vi "Remote Panel Multiple Client.vi"() -> ()   [LabVIEW 2024]
doc: "This VI illustrates how to programmatically connect to a remote front panel. A connection is established to the specified VI and control can also be requested. Once control is requested, the VI can only be run once since the server will close the connection automatically after one run."
panel:
  out "status":bool
  in  "Close Connection":bool
  in  "Open Connection":bool
  in  "Listbox":i32(listbox)
  in  "Stop":bool
  in  "Release Control":bool
  in  "Request Control":bool
  in  "RP Server Port":i32=8000
  in  "RP Server Address":string="localhost"
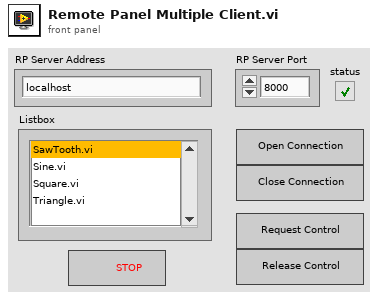
[diagram p1: front panel]
types:
  T1 = enum32{"invalid app kind", "Development System", "Run Time System", "Student Edition", "Embedded LabVIEW", "Evaluation", "Custom"}
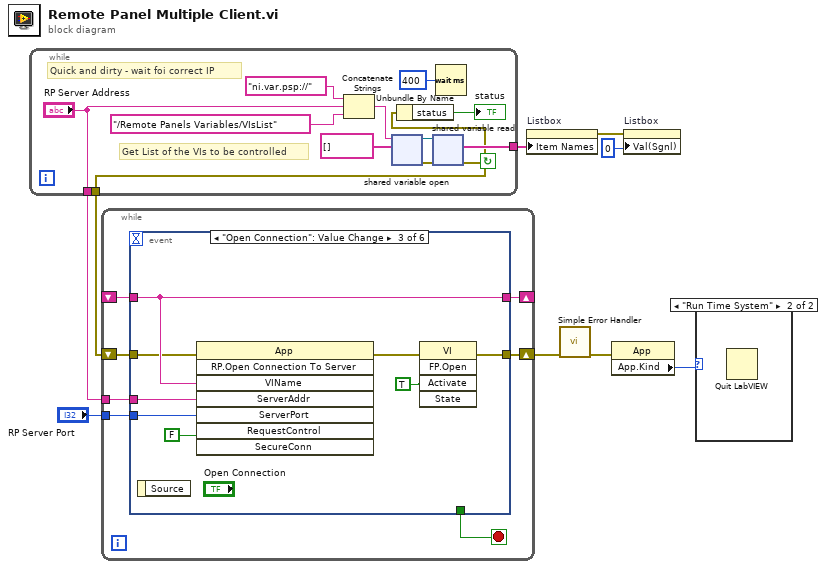
[diagram p0: block diagram]
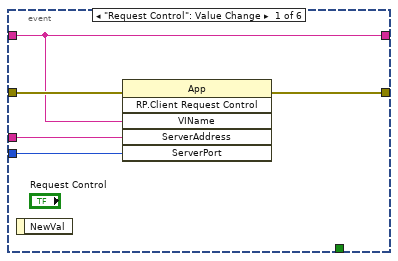
[diagram p3: hidden frame]
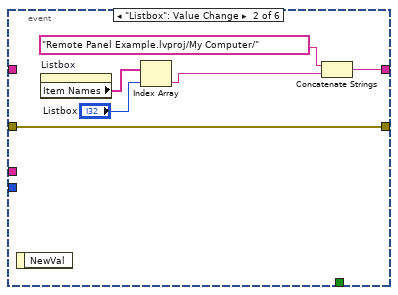
[diagram p4: hidden frame]
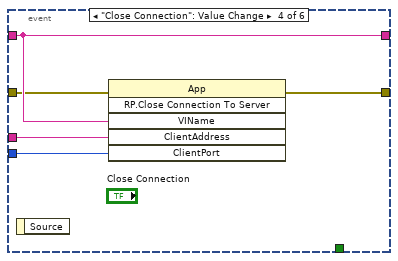
[diagram p5: hidden frame]
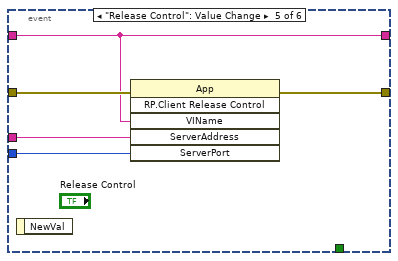
[diagram p6: hidden frame]
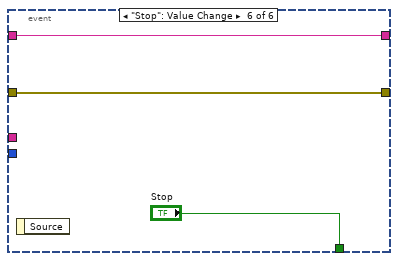
[diagram p7: hidden frame]
diagram:
  n1 = while {
    tunnel: [w17] -> w7
    tunnel: [w11] -> w6
    tunnel: ["RP Server Address"] -> w1
    stop <- w11 continue-if-true
    # "Quick and dirty - wait foi correct IP"
    # "Get List of the VIs to be controlled"
    n2 = Concatenate Strings("ni.var.psp://" ("string"), "RP Server Address", "/Remote Panels Variables/VIsList" ("/Remote Panels Variables/VIsList")) -> (w13:string)
    n3 = shared-variable-open(w13, string[] []) -> (w19:refnum<k21>, w18:errorcluster)  [unwired: 2 in]
    n4 = shared-variable-read(w19, w18) -> (w11:errorcluster, w17:string[])  [unwired: 2 out]
    n5 = Unbundle By Name(w11) -> ("status"=→"status":bool)
    n6 = Wait (ms)(milliseconds to wait=u32 400) -> ()  [unwired: 1 out]
  }
  n7 = while {
    tunnel: "RP Server Port" -> [w26]
    tunnel: w1 -> [w25]
    shift-right: [w27] -> w9
    shift-left: w6 -> [w24]
    shift-right: [w22] -> _
    shift-left: _ -> [w21]
    stop <- w23 stop-if-true
    n8 = event shown="[2] \"Open Connection\": Value Change" {
      selector: _ -> [_ _ _ _ _ _]
      dyn-events: _ -> [_ _ _ _ _ _]
      timeout: _ -> [_ _ _ _ _ _]
      tunnel: w24 -> [w32 w33 w40 w48 w56 w58]
      tunnel: [w31 w33 w39 w47 w55 w58] -> w27
      tunnel: w26 -> [w30 _ w42 w50 w54 _]
      tunnel: w25 -> [w29 _ w43 w51 w53 _]
      tunnel: [_ _ _ _ _ "Stop"] -> w23
      tunnel: [w28 w34 w41 w49 w52 w57] -> w22
      tunnel: w21 -> [w28 _ w41 w49 w52 w57]
      event "Request Control": Value Change {
        n9 = event-data() -> ()  [unwired: 1 in, 1 out]
        n10 = invoke class="App" method="RP.Client Request Control"(error in=w32, "VIName"=w28, "ServerAddress"=w29, "ServerPort"=w30) -> (error out=w31:errorcluster)  [unwired: 2 in, 5 out]
      }
      event "Listbox": Value Change {
        n11 = event-data() -> ()  [unwired: 1 in, 1 out]
        n12 = property on="Listbox" class="LstBox (strict)"() -> ("Item Names"=w38:string[])  [unwired: 2 in, 2 out]
        n13 = Index Array(array=w38, index="Listbox") -> (element=w36:string)
        n14 = Concatenate Strings("Remote Panel Example.lvproj/My Computer/" ("string"), w36) -> (w34:string)
      }
      event "Open Connection": Value Change {
        n15 = event-data() -> ()  [unwired: 1 in, 1 out]
        n16 = invoke class="App" method="RP.Open Connection To Server"(error in=w40, "VIName"=w41, "ServerAddr"=w43, "ServerPort"=w42, "RequestControl"=FALSE) -> (error out=w45:errorcluster)  [unwired: 3 in, 7 out]
        n17 = invoke class="VI" method="FP.Open"(error in=w45, "Activate"=TRUE ("Activate?")) -> (error out=w39:errorcluster)  [unwired: 3 in, 4 out]
      }
      event "Close Connection": Value Change {
        n18 = event-data() -> ()  [unwired: 1 in, 1 out]
        n19 = invoke class="App" method="RP.Close Connection To Server"(error in=w48, "VIName"=w49, "ClientAddress"=w51, "ClientPort"=w50) -> (error out=w47:errorcluster)  [unwired: 2 in, 5 out]
      }
      event "Release Control": Value Change {
        n20 = event-data() -> ()  [unwired: 1 in, 1 out]
        n21 = invoke class="App" method="RP.Client Release Control"(error in=w56, "VIName"=w52, "ServerAddress"=w53, "ServerPort"=w54) -> (error out=w55:errorcluster)  [unwired: 2 in, 5 out]
      }
      event "Stop": Value Change {
        n22 = event-data() -> ()  [unwired: 1 in, 1 out]
      }
    }
  }
  n23 = property on="Listbox" class="LstBox (strict)"("Item Names"=w7) -> (error out=w5:errorcluster)  [unwired: 2 in, 1 out]
  n24 = call <vilib>:"Simple Error Handler.vi"("error in (no error)"=w9) -> ("error out"=w3:errorcluster)  [unwired: 4 in, 4 out]
  n25 = property class="App"(error in=w3) -> ("App.Kind"=w2:T1)  [unwired: 1 in, 2 out]
  n26 = property on="Listbox" class="LstBox (strict)"(error in=w5, "Val(Sgnl)"=0 ("Value (Signaling)")) -> ()  [unwired: 1 in, 2 out]
  n27 = case shown="\"Run Time System\"" w2 {
    frame "invalid app kind", Default {
    }
    frame "Run Time System" {
      n28 = Quit LabVIEW() -> ()  [unwired: 1 in]
    }
  }
